vi "CNR abx reweighted.vi"(0 "parameters":dbl[](array[numeric]), 1 "model function":T4, 5 "method":T2 items=["Least Square", "Least Absolute Residual", "Bisquare"], 7 "scale factors":dbl[](array[numeric]), 9 "output control":T3={"model function"=TRUE, "gradient"=TRUE}, 11 "error in (no error)":errorcluster, 12 "Y":dbl[](array[numeric]), 13 "X":dbl[](array[numeric]), 14 "Weight":dbl[](array[numeric])) -> (2 "Jacobian":T1, 3 "number of function calls":i32, 4 "Hessian":T1, 6 "gradient":dbl[](array[numeric]), 8 "best fit":dbl[](array[numeric]), 10 "chiSqr":dbl, 15 "error out":errorcluster)   [LabVIEW 2017, in "NI_Gmath.lvlib"]
uses:
  <vilib>/gmath/NI_Gmath.lvlib
  <vilib>/Analysis/Matrix/Datatypes/RealMatrix.ctl
  <vilib>/gmath/NumericalOptimization/LM model function.ctl
  <vilib>/gmath/NumericalOptimization/LM model function reference.ctl
  <vilib>/gmath/NumericalOptimization/LM_output select.ctl
  <vilib>/Analysis/6fits.llb/Curve Fitting Criteria.ctl
  <vilib>/Analysis/baseanly.llb/Real Dot Product.vi
  <vilib>/Analysis/baseanly.llb/Real A x B.vi
  <vilib>/Analysis/baseanly.llb/A x Vector.vi
  <vilib>/Analysis/NI_AALBase.lvlib
  <vilib>/Analysis/Matrix/NI_Matrix.lvlib
  <vilib>/Analysis/NI_AALPro.lvlib
panel:
  # "Lev-Mar\nabx"
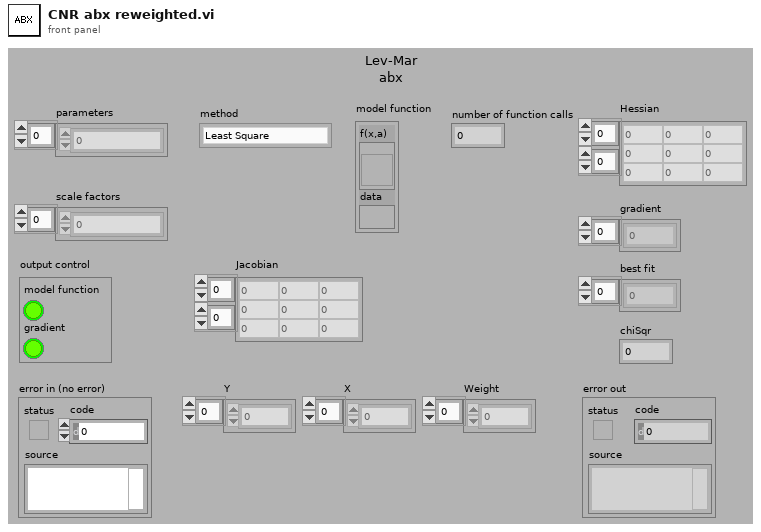
[diagram p1: front panel]
types:
  T1 = typedef "NI_Matrix.lvlib/RealMatrix.ctl" = dbl[][]
  T2 = typedef "NI_AALPro.lvlib/Curve Fitting Criteria.ctl" = u16
  T3 = typedef "NI_Gmath.lvlib/LM_output select.ctl" = cluster{"model function":bool, "gradient":bool}
  T4 = typedef "NI_Gmath.lvlib/LM model function.ctl" = cluster{"f(x,a)":T5, "data":variant}
  T5 = typedef "NI_Gmath.lvlib/LM model function reference.ctl" = refnum<vi>
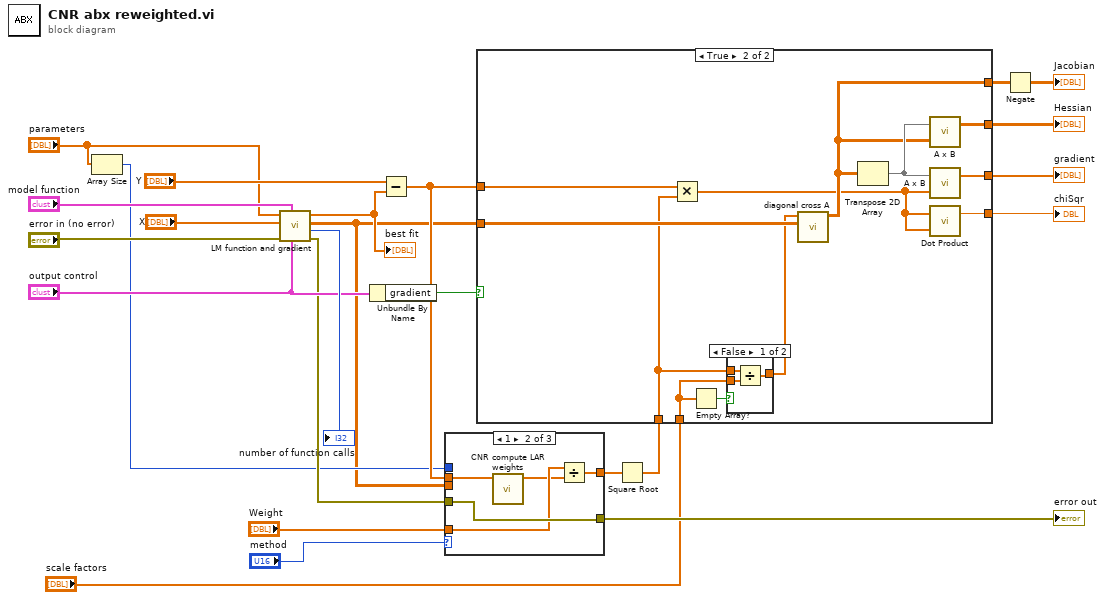
[diagram p0: block diagram]
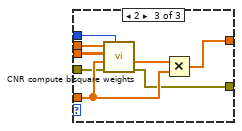
[diagram p3: hidden frame]
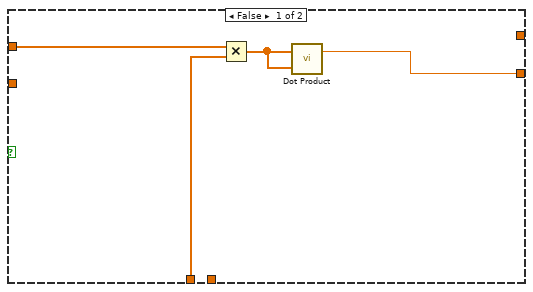
[diagram p4: hidden frame]
diagram:
  n1 = Array Size(array="parameters") -> (size(s)=w8:i32)
  n2 = call <vilib>:"LM function and gradient.vi"("output control"="output control", "model function"="model function", "error in (no error)"="error in (no error)", "X"="X", "a"="parameters") -> ("error out"=w16:errorcluster, "number of function calls"=→"number of function calls":i32, "gradient"=w3:dbl[][], "f(X)"=w18:dbl[])  [unwired: 3 out]
  "best fit" <- w18
  n3 = Unbundle By Name("output control") -> ("gradient"=w20:bool)
  n4 = Subtract(x="Y", y=w18) -> (x-y=w9:dbl[])
  n5 = case shown="1" "method" {
    tunnel: w3 -> [_ _ w39]
    tunnel: [w26 w29 w38] -> w5
    tunnel: "Weight" -> [w26 w30 w37]
    tunnel: [w25 w31 w36] -> w12
    tunnel: w16 -> [w25 w31 w35]
    tunnel: w9 -> [_ w28 w34]
    tunnel: w8 -> [_ _ w32]
    frame 0, Default {
    }
    frame 1 {
      n6 = call <vilib>:"CNR compute LAR weights.vi"("residuals"=w28) -> ("LAR weights"=w27:dbl[])  [unwired: 10 out]
      n7 = Divide(x=w30, y=w27) -> (x/y=w29:dbl[])
    }
    frame 2 {
      n8 = call <vilib>:"CNR compute bisquare weights.vi"("number of parameters"=w32, "error in (no error)"=w35, "weight"=w37, "J"=w39, "raw residuals"=w34) -> ("error out"=w36:errorcluster, "weights"=w33:dbl[])  [unwired: 5 out]
      n9 = Multiply(x=w33, y=w37) -> (x*y=w38:dbl[])
    }
  }
  "error out" <- w12
  n10 = Square Root(x=w5) -> (sqrt(x)=w6:dbl[])
  n11 = case shown="True" w20 {
    tunnel: [_ w45] -> w13
    tunnel: [_ w46] -> w1
    tunnel: [w40 w55] -> w24
    tunnel: w3 -> [_ w54]
    tunnel: w6 -> [w43 w51]
    tunnel: w9 -> [w42 w53]
    tunnel: "scale factors" -> [_ w49]
    tunnel: [_ w47] -> w2
    frame False {
      n12 = Multiply(x=w42, y=w43) -> (x*y=w41:dbl[])
      n13 = call-poly <vilib>:"Dot Product.vi"("Y Vector"=w41, "X Vector"=w41) -> ("X * Y"=w40:dbl)  [unwired: 1 out]
    }
    frame True {
      n14 = Multiply(x=w53, y=w51) -> (x*y=w44:dbl[])
      n15 = Empty Array?(array=w49) -> (empty?=w48:bool)
      n16 = case shown="False" w48 {
        tunnel: w51 -> [w58 w59]
        tunnel: w49 -> [w57 _]
        tunnel: [w56 w59] -> w50
        frame False {
          n17 = Divide(x=w58, y=w57) -> (x/y=w56:dbl[])
        }
        frame True {
        }
      }
      n18 = call <vilib>:"diagonal cross A.vi"("A"=w54, "diagonal"=w50) -> ("diagonalxA"=w47:T1)  [unwired: 9 out]
      n19 = Transpose 2D Array(2D array=w47) -> (transposed array=w52:T1)
      n20 = call-poly <vilib>:"A x B.vi"("B"=w47, "A"=w52) -> ("A x B"=w46:T1)  [unwired: 1 out]
      n21 = call-poly <vilib>:"A x B.vi"("Vector"=w44, "A"=w52) -> ("A x Vector"=w45:dbl[])  [unwired: 1 out]
      n22 = call-poly <vilib>:"Dot Product.vi"("Y Vector"=w44, "X Vector"=w44) -> ("X * Y"=w55:dbl)  [unwired: 1 out]
    }
  }
  "Hessian" <- w1
  "gradient" <- w13
  "chiSqr" <- w24
  n23 = Negate(x=w2) -> (-x=→"Jacobian":T1)
